vi "collision_plots.vi"(4 "error in":errorcluster, 7 "Collision sensor sample":string) -> (0 "error out":errorcluster, 3 "Collision Ocurred":bool)   [LabVIEW 2019, in "Lib_Simx.lvlib"]
doc: "Tool to plot the information provided by the collision sensor."
uses:
  Lib_Simx.lvlib
  controls/ncap.ctl
  controls/targets.ctl
panel:
  in  "Target to Plot":i32
  out "value":T1
  in  "Switch Tab":i32 min=0 max=10 step=1
  out "Tab Control":T3(tab)
  out "Acceleration GVT":cluster{"x":dbl, "y":dbl, "z":dbl}(graph)
  out "Acceleration":cluster{"x":dbl, "y":dbl, "z":dbl}(graph)
  out "Velocity":T4(graph)
  out "Distance":dbl(graph)
  out "Forward acceleration":T4(graph)
  out "TTC":dbl(graph)
  out "Throttle":T4(graph)
  out "Brake":T4(graph)
  out "Wheel":T4(graph)
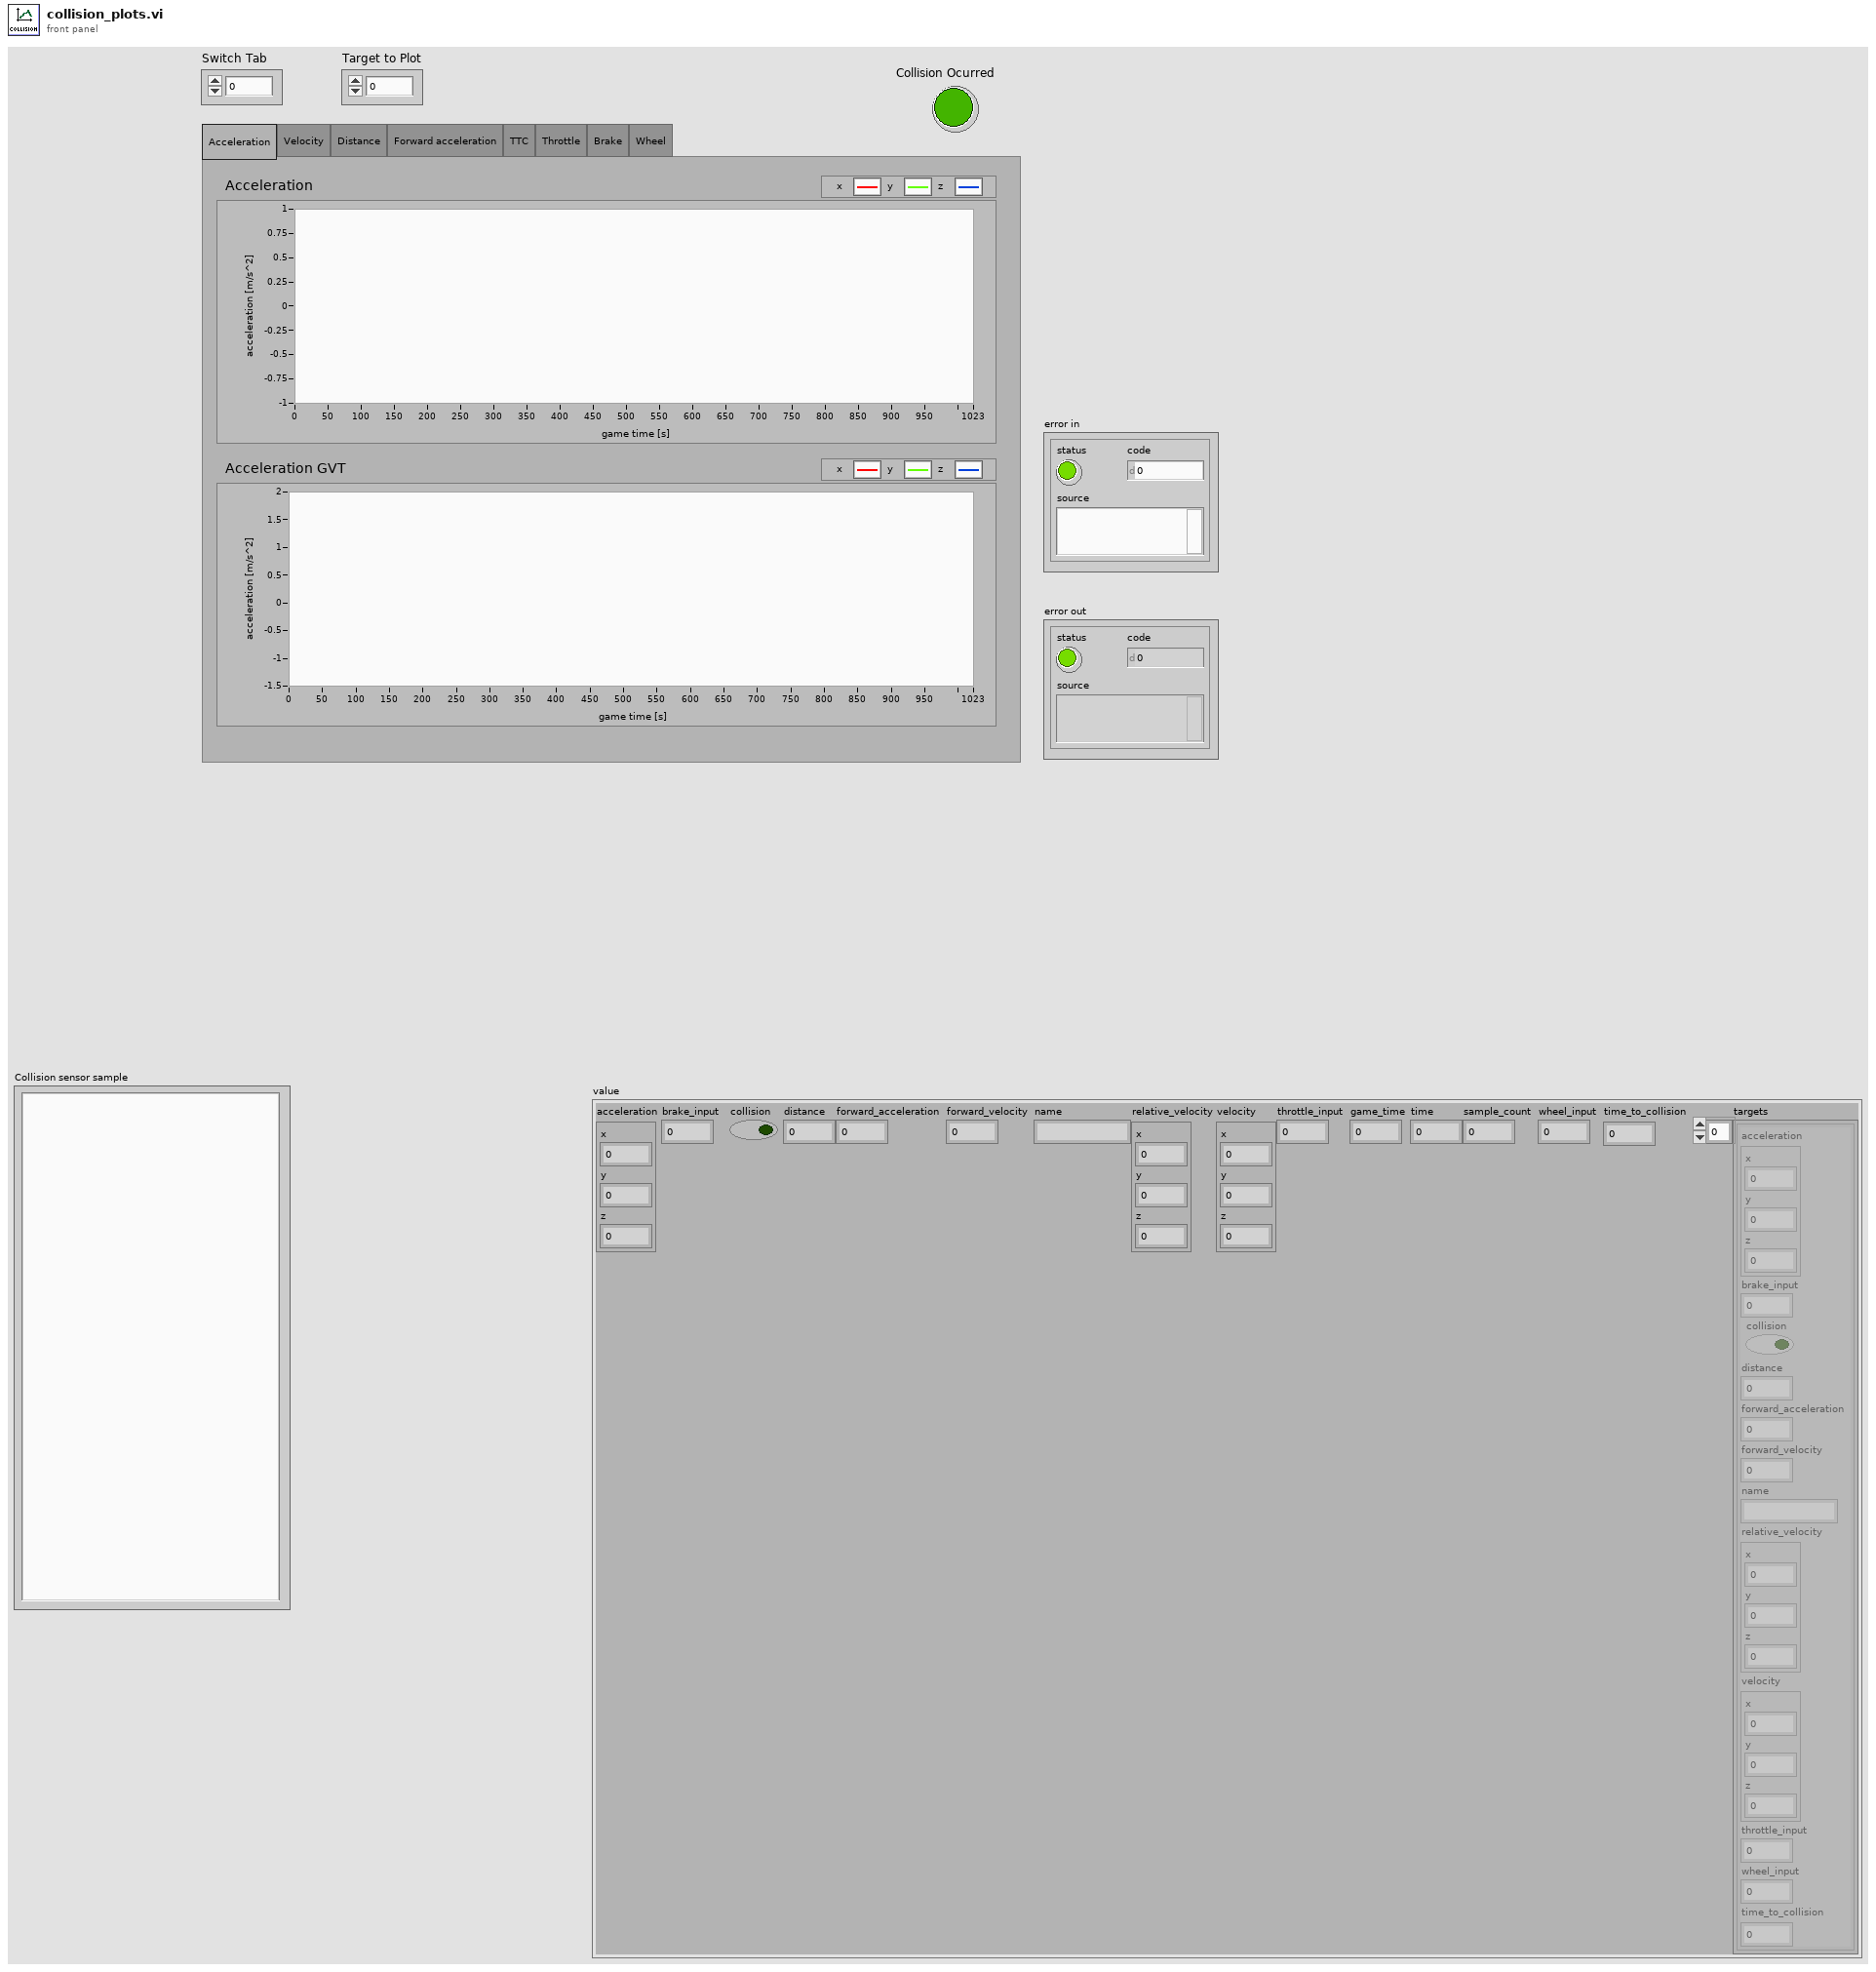
[diagram p1: front panel]
types:
  T1 = typedef "Lib_Simx.lvlib/ncap.ctl" = cluster{"acceleration":cluster{"x":dbl, "y":dbl, "z":dbl}, "brake_input":dbl, "collision":bool, "distance":dbl, "forward_acceleration":dbl, "forward_velocity":dbl, "name":string, "relative_velocity":cluster{"x":dbl, "y":dbl, "z":dbl}, "velocity":cluster{"x":dbl, "y":dbl, "z":dbl}, "throttle_input":dbl, "game_time":dbl, "time":dbl, "sample_count":i32, "wheel_input":dbl, "time_to_collision":dbl, "targets":T2[]}
  T2 = typedef "Lib_Simx.lvlib/targets.ctl" = cluster{"acceleration":cluster{"x":dbl, "y":dbl, "z":dbl}, "brake_input":dbl, "collision":bool, "distance":dbl, "forward_acceleration":dbl, "forward_velocity":dbl, "name":string, "relative_velocity":cluster{"x":dbl, "y":dbl, "z":dbl}, "velocity":cluster{"x":dbl, "y":dbl, "z":dbl}, "throttle_input":dbl, "wheel_input":dbl, "time_to_collision":dbl}
  T3 = enum32{"Acceleration", "Velocity", "Distance", "Forward acceleration", "TTC", "Throttle", "Brake", "Wheel"}
  T4 = cluster{"forward_velocity":dbl, "forward_velocity":dbl}
  T5 = cluster{"forward_velocity":dbl, "forward_velocity":dbl}[]
  T6 = cluster{"forward_acceleration":dbl, "forward_acceleration":dbl}
  T7 = cluster{"throttle_input":dbl, "throttle_input":dbl}
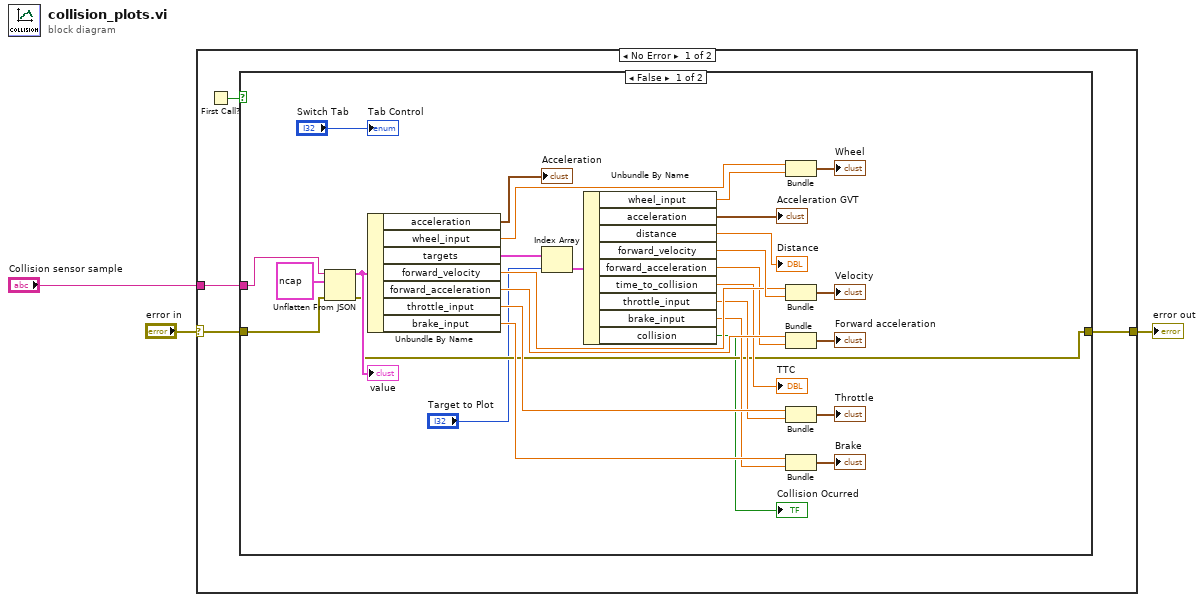
[diagram p0: block diagram]
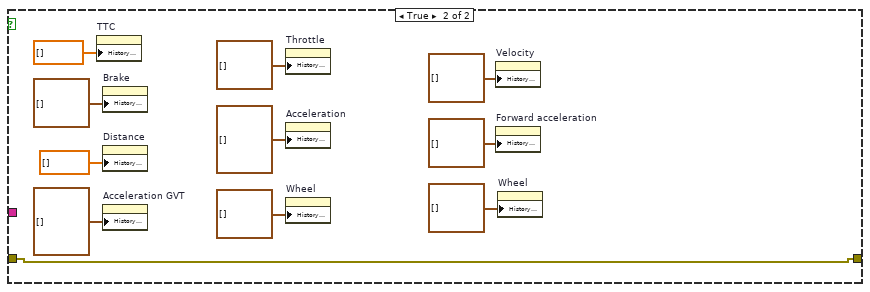
[diagram p2: hidden frame]
diagram:
  n1 = case shown="No Error" "error in" {
    selector: "error in" -> [w6 w48]
    tunnel: [w7 w48] -> w3
    tunnel: "Collision sensor sample" -> [w5 _]
    frame No Error {
      n2 = First Call?() -> (First Call?: T/F=w4:bool)
      n3 = case shown="False" w4 {
        tunnel: [w13 w45] -> w7
        tunnel: w6 -> [w12 w45]
        tunnel: w5 -> [w10 _]
        frame False {
          n4 = Unflatten From JSON(JSON string=w10, type and defaults=T1 {"acceleration"={"x"=0.0, "y"=0.0, "z"=0.0}, "brake_input"=0.0, "collision"=FALSE, "distance"=0.0, "forward_acceleration"=0.0, "forward_velocity"=0.0, "name"="", "relative_velocity"={"x"=0.0, "y"=0.0, "z"=0.0}, "velocity"={"x"=0.0, "y"=0.0, "z"=0.0}, "throttle_input"=0.0, "game_time"=0.0, "time"=0.0, "sample_count"=0, "wheel_input"=0.0, "time_to_collision"=0.0, "targets"=[]} ("ncap"), error in (no error)=w12) -> (value=w35:T1, error out=w13:errorcluster)  [unwired: 4 in]
          "value" <- w35
          n5 = Unbundle By Name(w35) -> ("acceleration"=→"Acceleration":cluster{"x":dbl, "y":dbl, "z":dbl}, "wheel_input"=w32:dbl, "targets"=w34:T2[], "forward_velocity"=w25:dbl, "forward_acceleration"=w24:dbl, "throttle_input"=w20:dbl, "brake_input"=w17:dbl)
          n6 = Index Array(array=w34, index="Target to Plot") -> (element=w33:T2)
          n7 = Unbundle By Name(w33) -> ("wheel_input"=w31:dbl, "acceleration"=→"Acceleration GVT":cluster{"x":dbl, "y":dbl, "z":dbl}, "distance"=→"Distance":dbl, "forward_velocity"=w26:dbl, "forward_acceleration"=w23:dbl, "time_to_collision"=→"TTC":dbl, "throttle_input"=w19:dbl, "brake_input"=w16:dbl, "collision"=→"Collision Ocurred":bool)
          n8 = Bundle("wheel_input"=w32, "wheel_input"=w31) -> (→"Wheel":cluster{"wheel_input":dbl, "wheel_input":dbl})  [unwired: 1 in]
          n9 = Bundle("forward_velocity"=w25, "forward_velocity"=w26) -> (→"Velocity":T4)  [unwired: 1 in]
          n10 = Bundle("forward_acceleration"=w24, "forward_acceleration"=w23) -> (→"Forward acceleration":T6)  [unwired: 1 in]
          n11 = Bundle("throttle_input"=w20, "throttle_input"=w19) -> (→"Throttle":T7)  [unwired: 1 in]
          n12 = Bundle("brake_input"=w17, "brake_input"=w16) -> (→"Brake":cluster{"brake_input":dbl, "brake_input":dbl})  [unwired: 1 in]
          "Tab Control" <- "Switch Tab"
        }
        frame True {
          n13 = property on="TTC" class="WFChart (strict)"("History Data"=dbl[] []) -> ()  [unwired: 2 in, 2 out]
          n14 = property on="Brake" class="WFChart (strict)"("History Data"=T5 []) -> ()  [unwired: 2 in, 2 out]
          n15 = property on="Distance" class="WFChart (strict)"("History Data"=dbl[] []) -> ()  [unwired: 2 in, 2 out]
          n16 = property on="Acceleration GVT" class="WFChart (strict)"("History Data"=cluster{"x":dbl, "y":dbl, "z":dbl}[] []) -> ()  [unwired: 2 in, 2 out]
          n17 = property on="Throttle" class="WFChart (strict)"("History Data"=T5 []) -> ()  [unwired: 2 in, 2 out]
          n18 = property on="Acceleration" class="WFChart (strict)"("History Data"=cluster{"x":dbl, "y":dbl, "z":dbl}[] []) -> ()  [unwired: 2 in, 2 out]
          n19 = property on="Wheel" class="WFChart (strict)"("History Data"=T5 []) -> ()  [unwired: 2 in, 2 out]
          n20 = property on="Velocity" class="WFChart (strict)"("History Data"=T5 []) -> ()  [unwired: 2 in, 2 out]
          n21 = property on="Forward acceleration" class="WFChart (strict)"("History Data"=T5 []) -> ()  [unwired: 2 in, 2 out]
          n22 = property on="Wheel" class="WFChart (strict)"("History Data"=T5 []) -> ()  [unwired: 2 in, 2 out]
        }
      }
    }
    frame Error {
    }
  }
  "error out" <- w3
